vi "WGO.vi"(0 "System no.":i32=1 min=1 max=4 step=1, 2 "Affected axes":string[](array[string]), 3 "WGO Parameter":i32[](array[numeric]), 5 "error in":errorcluster) -> (14 "Controller error":bool, 19 "error out":errorcluster)   [LabVIEW 2020]
doc: "Enables, disables, and sets wave generator output mode. Parameter is bit-mapped. Controller error is TRUE if selected system reports an error code which is not zero.\n\nC-413: Affected axis is identical with wave generator number, which can be 1 to 2. See C-413 user manual for a description of valid parameters. Use DRC to configure data recording. Recording ends when the record table content has reached the maximum number of points (4096 in total). Starting the wave generator is not allowed when the analog input is used for target generation.\n\nC-886: Affected axis is identical with wave generator number, which can be 1 to No. of connected axes. See controller user manual for a description of valid parameters. Recording ends when the record table content has reached the maximum number of points (1 Million in total). Starting the wave generator is not allowed when axes are moving. \n\nC-887: Affected axis is identical with wave generator number, which can be 1 to No. of connected axes. See controller user manual for a description of valid parameters.Use DRC to configure data recording. Recording ends when the record table content has reached the maximum number of points (4 Million in total). Starting the wave generator is not allowed when axes are moving. \n\nC-891: Affected axis is identical with wave generator number, which can be 1. See controller user manual for a description of valid parameters.Use DRC to configure data recording. Recording ends when the record table content has reached the maximum number of points (16384 in total).\n\nE-516: See user manual for parameter definition.\n\nE-517, E-518: Affected axis is identical with wave generator number, which can be 1 to 3. See controller user manual for a description of valid parameters. Use DRC to configure data recording. Recording ends when the record table content has reached the maximum number of points (8,192 in total).\n\nE-709: Affected axis is identical with wave generator number, which can be 1.See E-709 user manual for a description of valid parameters. Use DRC to configure data recording. Recording ends when the record table content has reached the maximum number of points (4096 in total). Starting the wave generator is not allowed when the analog input is used for target generation.\n\nE-710: Affected axis is identical with wave generator number. Only two wave generators can run simultaneously. See E7XX_GCS_DLL Manual for parameter definition.\n\nE-712: Affected axis is identical with wave generator number, which can be 1 to No. of connected axes.See E-712 user manual for a description of valid parameters. Use DRC to configure data recording. Recording ends when the record table content has reached the maximum number of points (262,144 in total). Starting the wave generator is not allowed when the analog input is used for target generation.\n\nE-725: Affected axis is identical with wave generator number, which can be 1 to 3. See E-725 user manual for a description of valid parameters. Use DRC to configure data recording. Recording ends when the record table content has reached the maximum number of points (262,144 in total). Starting the wave generator is not allowed when the analog input is used for target generation.\n\nE-727: Affected axis is identical with wave generator number, which can be 1 to 4. See E-727 user manual for a description of valid parameters.Use DRC to configure data recording. Recording ends when the record table content has reached the maximum number of points (262,144 in total). Starting the wave generator is not allowed when the analog input is used for target generation.\n\nE-753: Affected axis is identical with wave generator number, which can be 1. See E-753 user manual for a description of valid parameters. Use DRC to configure data recording. Recording ends when the record table content has reached the maximum number of points (65,536 in total). Starting the wave generator is not allowed when the analog input is used for target generation.\n\nE-754: Affected axis is identical with wave generator number, which can be 1. See controller user manual for a description of valid parameters. Use DRC to configure data recording. Recording ends when the record table content has reached the maximum number of points (1,048,576 in total). Starting the wave generator is not allowed when the analog input is used for target generation.\n\nE-761: Affected axis is identical with wave generator number, which can be 1 to 4. Four wave generators can run simultaneously. See E7XX_GCS_DLL Manual for parameter definition. Each time the wave generator is started recording starts automatically as follows: recorder table 1: axis 1 actual position, recorder table 2: axis 2 actual position, recorder table 3: axis 3 actual position, recorder table 4: analog input voltage (same value as read with TAV?.vi, i.e. contains gain and offset for the analog input, see E-761 user manual. Recording ends when the record table content has reached the maximum number of points (8192 per table)."
panel:
  # "Enables, disables and sets wave generator output mode. Parameter\nis bit-mapped."
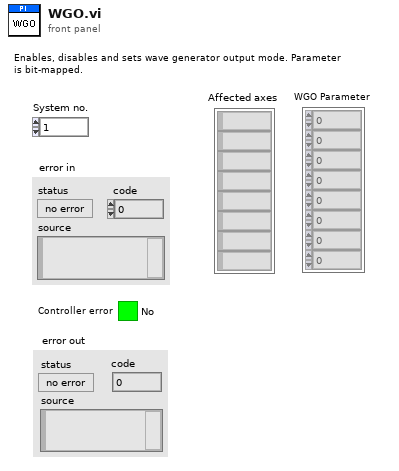
[diagram p1: front panel]
types:
  T1 = enum16{"Disable error check", "Force error check", "Use global settings"}
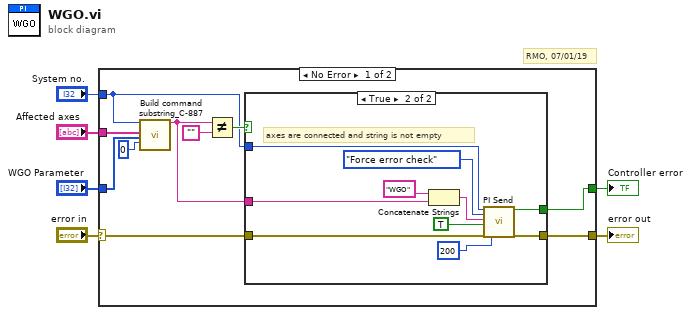
[diagram p0: block diagram]
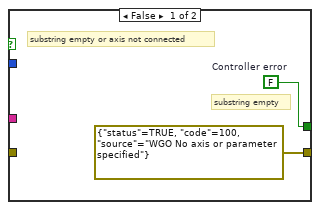
[diagram p2: hidden frame]
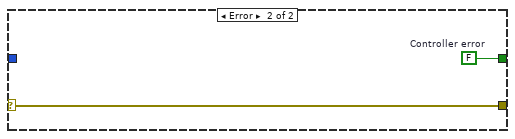
[diagram p3: hidden frame]
diagram:
  # "RMO, 07/01/19"
  n1 = case shown="No Error" "error in" {
    selector: "error in" -> [w8 w30]
    tunnel: [w16 w30] -> w6
    tunnel: "WGO Parameter" -> [w13 _]
    tunnel: "System no." -> [w9 _]
    tunnel: "Affected axes" -> [w12 _]
    tunnel: [w7 w29] -> w1
    frame No Error {
      n2 = call "Build command substring_C-887.vi"("System no."=w9, "Affected axes"=w12, "Parameters"=w13, "No. of digits"=i16 0 ("No.of digits")) -> ("Command substring"=w14:string)  [unwired: 3 in, 12 out]
      n3 = Not Equal?(x=w14, y="") -> (x != y?=w10:bool)
      n4 = case shown="True" w10 {
        tunnel: w14 -> [_ w27]
        tunnel: [errorcluster {"status"=TRUE, "code"=100, "source"="WGO No axis or parameter specified"} ("error out") w21] -> w16
        tunnel: w8 -> [_ w24]
        tunnel: w9 -> [_ w23]
        tunnel: [w17 w20] -> w7
        frame False {
          w17 = FALSE  # Controller error
          # "substring empty"
          # "substring empty or axis not connected"
        }
        frame True {
          # "axes are connected and string is not empty"
          n5 = Concatenate Strings("WGO", w27) -> (w25:string)
          n6 = call "PI Send.vi"("System no."=w23, "Error check settings"=T1."Force error check", "String to send"=w25, "Attach termination char.?"=TRUE ("Attach Linefeed?"), "error in"=w24, "Delay before error check (ms)"=u32 200 ("milliseconds to wait")) -> ("Controller error"=w20:bool, "error out"=w21:errorcluster)  [unwired: 12 out]
        }
      }
    }
    frame Error {
      w29 = FALSE  # Controller error
    }
  }
  "error out" <- w6
  "Controller error" <- w1
